vi "Player Info.vi"(8 "Victory Speech":string="All your base are belong to us!!", 9 "Name":string="Sleepy Engineer", 11 "Formics in":refnum<class "Formics.lvclass">) -> (3 "Formics out":refnum<class "Formics.lvclass">)   [LabVIEW 2015, in "Formics.lvclass"]
uses:
  Formics.lvclass
  Square/Square.lvclass
panel:
  # "Set default values for these two string controls"
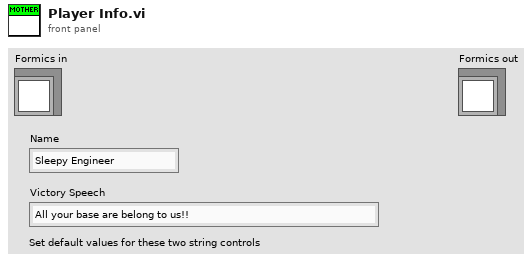
[diagram p1: front panel]
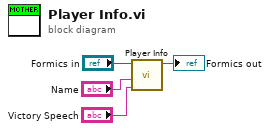
[diagram p0: block diagram]
diagram:
  n1 = call-parent "Player Info.vi"("Victory Speech"="Victory Speech", "Name"="Name", "Square in"="Formics in") -> ("Square out"=→"Formics out":refnum<class "Formics.lvclass">)  [unwired: 8 in]
